vi "RT_Main.vi"() -> ()   [LabVIEW 2019]
uses:
  <vilib>/myRIO/Instrument Drivers/Onboard IO/DIO/typedefs/DIO Reference.ctl
  <vilib>/myRIO/Common/Instrument Driver Framework/Utilities/typedefs/myRIO Generic Hardware Reference.ctl
  <vilib>/myRIO/Common/Instrument Driver Framework/Utilities/typedefs/Hardware Version Enum.ctl
  <vilib>/myRIO/Common/Instrument Driver Framework/Utilities/typedefs/myRIO v1.0 Reference.ctl
  <vilib>/myRIO/Common/Instrument Driver Framework/Utilities/typedefs/Generic FPGA Reference.ctl
  <vilib>/myRIO/Common/Instrument Driver Framework/myRIO v1.0/DIO/typedefs/DIO Channels List.ctl
  <vilib>/myRIO/Common/Instrument Driver Framework/myRIO v1.0/DIO/typedefs/DIO Channels Enum.ctl
  <vilib>/userdefined/High Color/nirio_resource_hc.ctl
  <vilib>/myRIO/Instrument Drivers/Onboard IO/I2C/typedefs/I2C User Configuration.ctl
  <vilib>/myRIO/Instrument Drivers/Onboard IO/I2C/typedefs/I2C Transfer Rate.ctl
  <vilib>/myRIO/Instrument Drivers/Onboard Devices/Accelerometer/typedefs/Accelerometer Reference.ctl
  <vilib>/myRIO/Common/Instrument Driver Framework/myRIO v1.0/Accelerometer/typedefs/Accelerometer Channels List.ctl
  <vilib>/myRIO/Common/Instrument Driver Framework/myRIO v1.0/Accelerometer/typedefs/Accelerometer Channels Enum.ctl
  <vilib>/myRIO/Common/Instrument Driver Framework/Utilities/vis/Is FPGA Ref Available.vi
  <vilib>/myRIO/Common/Instrument Driver Framework/myRIO v1.0/DIO/vis/myRIO v1.1 Open DIO.vi
  <vilib>/myRIO/Common/Instrument Driver Framework/myRIO v1.0/Accelerometer/vis/myRIO v1.1 Open Accelerometer.vi
  <vilib>/myRIO/Common/Instrument Driver Framework/Utilities/vis/Validate Channels.vi
  <vilib>/myRIO/Common/Instrument Driver Framework/myRIO v1.0/DIO/vis/myRIO v1.0 Reserve DIO.vi
  <vilib>/myRIO/Common/Instrument Driver Framework/myRIO v1.0/I2C/vis/myRIO v1.0 Close I2C.vi
  <vilib>/myRIO/Common/Instrument Driver Framework/myRIO v1.0/Accelerometer/vis/myRIO v1.0 Reserve Accelerometer.vi
  <vilib>/myRIO/Common/Instrument Driver Framework/myRIO v1.0/UART/vis/myRIO v1.0 Close UART.vi
  <vilib>/myRIO/Common/Instrument Driver Framework/myRIO v1.0/Resource Manager/vis/myRIO v1.0 Reserve Channel List.vi
  <vilib>/myRIO/Common/Instrument Driver Framework/myRIO v1.0/DIO/vis/myRIO v1.0 Build MUX Configuration DIO.vi
  <vilib>/myRIO/Common/Instrument Driver Framework/myRIO v1.0/I2C/vis/myRIO v1.0 Unreserve I2C.vi
  <vilib>/myRIO/Common/Instrument Driver Framework/myRIO v1.0/Accelerometer/vis/myRIO v1.0 Build MUX Configuration Accelerometer.vi
  <vilib>/myRIO/Common/Instrument Driver Framework/myRIO v1.0/Resource Manager/vis/myRIO v1.0 Reserve Channel.vi
  <vilib>/myRIO/Common/Instrument Driver Framework/myRIO v1.0/Resource Manager/vis/myRIO v1.0 Unreserve Channel.vi
  <vilib>/myRIO/Common/Instrument Driver Framework/myRIO v1.0/Resource Manager/vis/myRIO v1.0 Create Configuration List.vi
  <vilib>/myRIO/Common/Instrument Driver Framework/myRIO v1.0/I2C/vis/myRIO v1.0 Build MUX Configuration I2C.vi
  <vilib>/myRIO/Common/Instrument Driver Framework/myRIO v1.0/Resource Manager/vis/myRIO v1.0 Unreserve Channel List.vi
  <vilib>/myRIO/Common/Instrument Driver Framework/myRIO v1.0/Resource Manager/vis/myRIO v1.0 Build Mutex Name.vi
  <vilib>/functionblocks/Counter/Elapsed Timer/Elapsed Timer.vi
  <vilib>/Utility/VariantDataType/GetNumericInfo.vi
  <vilib>/Utility/error.llb/Error Cluster From Error Code.vi
  <vilib>/myRIO/Common/Instrument Driver Framework/myRIO v1.0/myRIO v1.1 Open.vi
  <vilib>/myRIO/Common/Instrument Driver Framework/Utilities/vis/IO Manager.vi
  <vilib>/myRIO/Common/Instrument Driver Framework/Utilities/vis/Configuration Manager.vi
  <vilib>/myRIO/Common/Instrument Driver Framework/myRIO v1.0/Resource Manager/vis/myRIO v1.0 Configure IO.vi
  <vilib>/myRIO/Common/Instrument Driver Framework/myRIO v1.0/myRIO v1.0 Close.vi
  <vilib>/myRIO/Common/Instrument Driver Framework/myRIO v1.0/DIO/vis/myRIO v1.0 Read DIO.vi
  <vilib>/myRIO/Common/Instrument Driver Framework/myRIO v1.0/PWM/vis/myRIO v1.0 Write PWM.vi
  <vilib>/myRIO/Common/Instrument Driver Framework/myRIO v1.0/DIO/vis/myRIO v1.0 Write DIO.vi
  <vilib>/myRIO/Common/Instrument Driver Framework/myRIO v1.0/Accelerometer/vis/myRIO v1.0 Get Scaling Constant Accelerometer.vi
  <vilib>/myRIO/Common/Instrument Driver Framework/myRIO v1.0/Accelerometer/vis/myRIO v1.0 Read Accelerometer.vi
  <vilib>/myRIO/Common/Instrument Driver Framework/myRIO v1.0/I2C/vis/myRIO v1.0 Configure I2C.vi
  <vilib>/myRIO/Common/Instrument Driver Framework/myRIO v1.0/I2C/vis/myRIO v1.0 Shutdown I2C.vi
  <vilib>/myRIO/Common/Instrument Driver Framework/myRIO v1.0/AI/vis/myRIO v1.0 Read AI.vi
  <vilib>/myRIO/Common/Instrument Driver Framework/Utilities/vis/FPGA Ref Manager.vi
  <vilib>/myRIO/Common/Instrument Driver Framework/myRIO v1.0/myRIO v1.0 Reset FPGA.vi
  <vilib>/myRIO/Common/Instrument Driver Framework/myRIO v1.0/IRQ/vis/myRIO v1.0 IRQ Info FGV.vi
  <vilib>/myRIO/Common/Instrument Driver Framework/myRIO v1.0/IRQ/vis/myRIO v1.0 Timer IRQ Info FGV.vi
  <vilib>/myRIO/Common/Instrument Driver Framework/myRIO v1.0/IRQ/vis/myRIO v1.0 ISR Agent.vi
  <vilib>/myRIO/Instrument Drivers/Utilities/vis/Reset Index.vi
  <vilib>/myRIO/Common/Instrument Driver Framework/myRIO v1.0/Resource Manager/vis/myRIO v1.0 Block Write Resource Manager.vi
  <vilib>/functionblocks/FB Core/FB Core.xnode
  <vilib>/myRIO/Express VI/Onboard IO/DI/DI Express VI.xnode
  <vilib>/myRIO/Instrument Drivers/Onboard IO/DIO/vis/myRIO DIO Open.xnode
  <vilib>/myRIO/Express VI/Onboard Devices/Accelerometer/Accelerometer Express VI.xnode
  <vilib>/myRIO/Instrument Drivers/Onboard Devices/Accelerometer/vis/myRIO Accelerometer Open.xnode
  <vilib>/myRIO/Express VI/Onboard IO/DO/DO Express VI.xnode
  <vilib>/myRIO/Instrument Drivers/Onboard IO/I2C/I2C.lvlib
  <vilib>/myRIO/Instrument Drivers/Onboard IO/AI/AI.lvlib
  <vilib>/myRIO/Instrument Drivers/Utilities/Utilities.lvlib
  <vilib>/functionblocks/NI_FunctionBlock Libraries.lvlib
  <vilib>/myRIO/Instrument Drivers/Onboard IO/DIO/DIO.lvlib
  <vilib>/myRIO/Instrument Drivers/Onboard IO/PWM/PWM.lvlib
  <vilib>/myRIO/Instrument Drivers/Onboard Devices/Accelerometer/Accelerometer.lvlib
panel:
  out "Time":dbl
  out "X-Axis":dbl=-0.00390625
  out "Y-Axis":dbl=-0.1171875
  out "Z-Axis":dbl=0.98046875
  in  "Tab Control":T1(tab)
  out "Cluster":T2
  in  "Tab Control 3":enum32{"Simple", "Advanced"}(tab)
  in  "Up Button":bool
  in  "Down Button":bool
  in  "Enable":bool
  in  "Direction":bool
  out "Accelerometer Readings":T2(graph)={"X-Axis"=-0.00390625, "Y-Axis"=-0.1171875, "Z-Axis"=0.98046875}
  out "GPS Time":string
  in  "Air Sample":bool
  in  "Log File Name":string="LocationLog"
  in  "Sampler Step Freq":dbl(slide)=253.06122448979593 scale=100.0..300.0
  out "Storage Status":string=" 34.4 GB capacity with 25.7 GB free (74.8%)"
  in  "Plot Reset":bool
  out "Latitude":dbl=0.03333333333333333
  out "Longitude":dbl=0.050000555555555555
  out "Speed":dbl
  out "GPS Location":cluster{dbl[], dbl[]}(graph)
  out "IR Distance Left":dbl=740.0516187067414 format="%#3_4g"
  out "IR Distance Right":dbl=1850.783507510213 format="%#_4g"
  out "Sonar Distance":dbl=80.530998125 format="%#_4g"
  in  "Stop button":bool
  in  "Log Data?":bool=TRUE
  out "Logging Error Out":errorcluster
  out "File storage error out":errorcluster
  out "error IO":errorcluster
  out "Accelerometer Error Out":errorcluster
  out "Initialize Error Out":errorcluster={"status"=FALSE, "code"=-1950679034, "source"="Shared Variable in RT_Main.vi<APPEND>\nThis error or warning occurred while reading the following Shared Variable:\n\\\\OSoleRIO\\Target Library\\SonarDistance\n\\\\172.16.0.1\\Target Library\\SonarDistance"}
  out "Initialization Timed Out?":bool
  out "Main":i32=272259
  out "GPS":i32=1046
  out "IR":i32=5434
  out "Sonar":i32=2765
  out "UI":i32=25031
  out "Motor":i32=299489
  out "Logging":i32=126701
  out "Storage Status 2":i32=558
  out "Accelerometer":i32
  in  "Time zone":i32=1
  # "Soil Sample"
  # "True=Up False=Down"
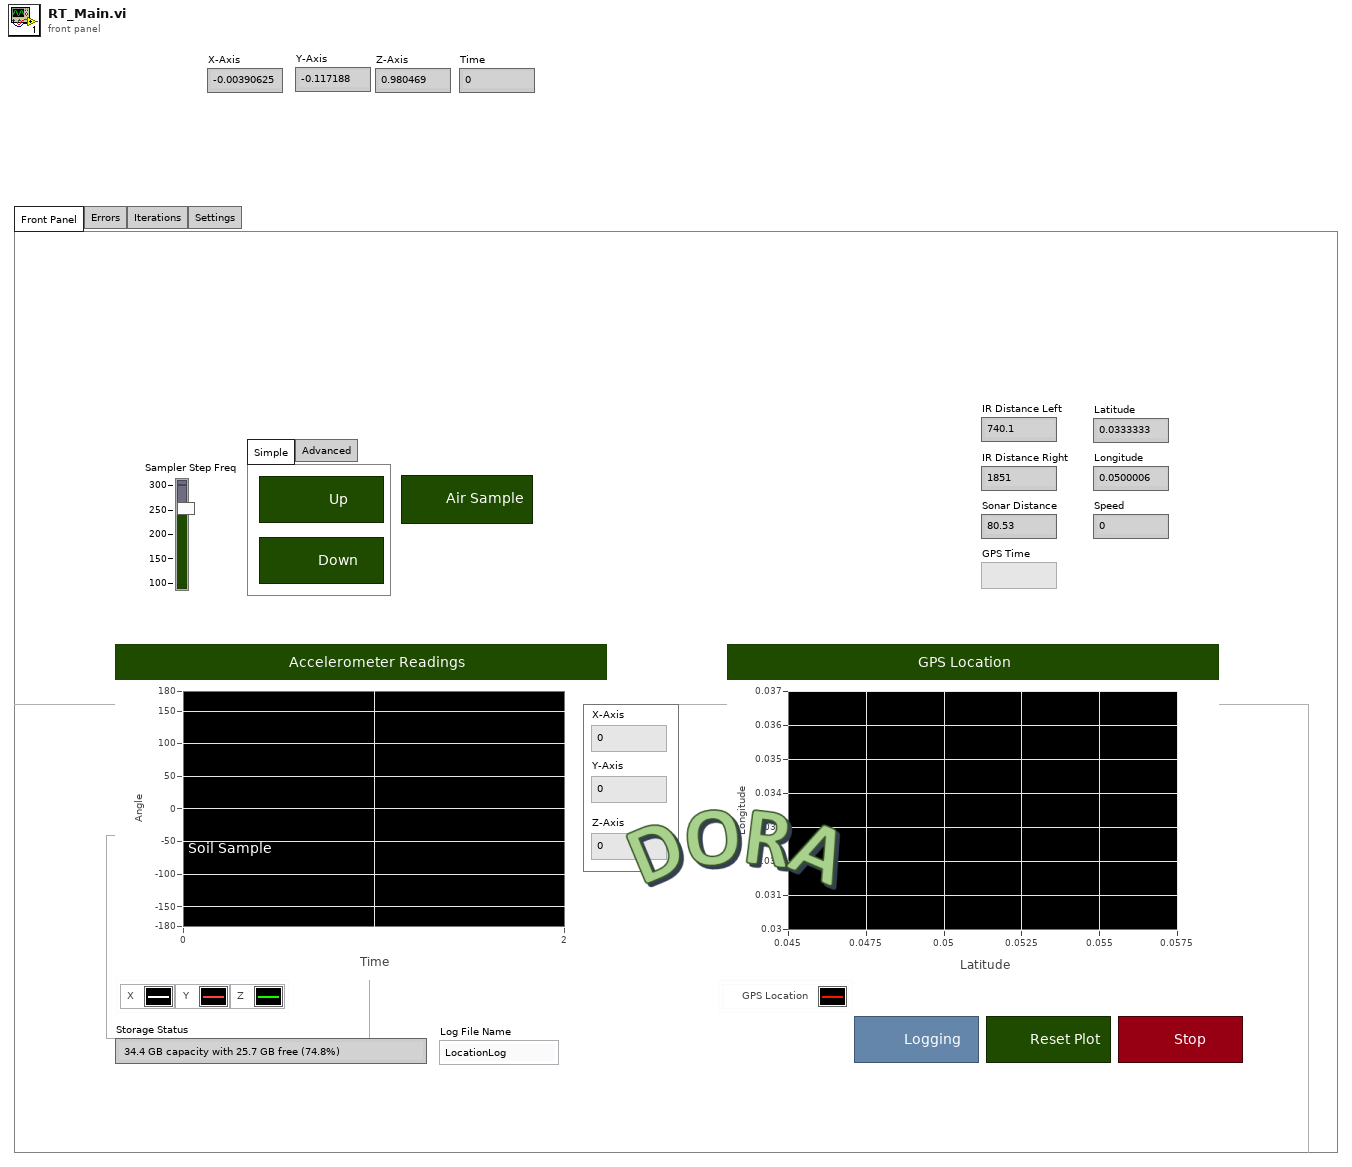
[diagram p1: front panel]
types:
  T1 = enum32{"Front Panel", "Errors", "Iterations", "Settings"}
  T2 = cluster{"X-Axis":dbl, "Y-Axis":dbl, "Z-Axis":dbl}
  T3 = enum16{"open", "replace", "create", "open or create", "replace or create", "replace or create with confirmation"}
  T4 = typedef "DIO.lvlib/DIO Reference.ctl" = cluster{"myRIO Reference":T5, "DIO Channels List":T9}
  T5 = typedef "myRIO Generic Hardware Reference.ctl" = cluster{"myRIO Model":T6, "myRIO Hardware Reference":T7}
  T6 = typedef "Hardware Version Enum.ctl" = enum16{"Unknown", "myRIO-1900", "myRIO-1950", "roboRIO", "NI ELVIS RIO CM", "ELVIS III"}
  T7 = typedef "myRIO v1.0 Reference.ctl" = cluster{"Generic FPGA Reference":T8, "Allow multiple opens":bool}
  T8 = typedef "Generic FPGA Reference.ctl" = refnum<k20>
  T9 = typedef "DIO Channels List.ctl" = T10[]
  T10 = typedef "DIO Channels Enum.ctl" = enum16{"Not Connected", "C/DIO0", "C/DIO1", "C/DIO2", "C/DIO3", "C/DIO4", "C/DIO5", "C/DIO6", "C/DIO7", "A/DIO0", "A/DIO1", "A/DIO2", "A/DIO3", "A/DIO4", "A/DIO5", "A/DIO6", "A/DIO7", "A/DIO8", "A/DIO9", "A/DIO10", "A/DIO11", "A/DIO12", "A/DIO13", "A/DIO14", "A/DIO15", "A/DIO16", "A/DIO17", "A/DIO18", "A/DIO19", "B/DIO0", "B/DIO1", "B/DIO2", "B/DIO3", "B/DIO4", "B/DIO5", "B/DIO6", "B/DIO7", "B/DIO8", "B/DIO9", "B/DIO10", "B/DIO11", "B/DIO12", "B/DIO13", "B/DIO14", "B/DIO15", "B/DIO16", "B/DIO17", "B/DIO18", "B/DIO19", "LED0", "LED1", "LED2", "LED3", "Button0", "DIO/DIO0", "DIO/DIO1", "DIO/DIO2", "DIO/DIO3", "DIO/DIO4", "DIO/DIO5", "DIO/DIO6", "DIO/DIO7", "DIO/DIO8", "DIO/DIO9", "SPI/CS0", "SPI/CS1", "SPI/CS2", "SPI/CS3", "LED RADIO (Green)", "LED RADIO (Red)", "LED COMM (Green)", "LED COMM (Red)", "LED MODE (Green)", "LED MODE (Red)"}
  T11 = typedef "nirio_resource_hc.ctl" = tag
  T12 = typedef "I2C.lvlib/I2C User Configuration.ctl" = cluster{"I2C Transfer Rate":T13}
  T13 = typedef "I2C.lvlib/I2C Transfer Rate.ctl" = enum16{"Standard mode (100 kbps)", "Fast mode (400 kbps)"}
  T14 = typedef "Accelerometer.lvlib/Accelerometer Reference.ctl" = cluster{"myRIO Reference":T5, "Accelerometer Channels List":T15, "LSB Weight":dbl}
  T15 = typedef "Accelerometer Channels List.ctl" = T16[]
  T16 = typedef "Accelerometer Channels Enum.ctl" = enum16{"Not Connected", "X-Axis", "Y-Axis", "Z-Axis"}
  T17 = typedef "AI.lvlib/AI Reference.ctl" = cluster{"myRIO Reference":T5, "AI Channels List":T18, "AI Scaling Constants List":T20}
  T18 = typedef "AI Channels List.ctl" = T19[]
  T19 = typedef "AI Channels Enum.ctl" = enum16{"Not Connected", "AudioIn/Left", "AudioIn/Right", "C/AI0", "C/AI1", "A/AI0", "A/AI1", "A/AI2", "A/AI3", "A/AI4", "A/AI5", "A/AI6", "A/AI7", "B/AI0", "B/AI1", "B/AI2", "B/AI3", "B/AI4", "B/AI5", "B/AI6", "B/AI7", "AI/AI0", "AI/AI1", "AI/AI2", "AI/AI3", "A/AI0 (DIFF)", "A/AI1 (DIFF)", "A/AI2 (DIFF)", "A/AI3 (DIFF)", "B/AI0 (DIFF)", "B/AI1 (DIFF)", "B/AI2 (DIFF)", "B/AI3 (DIFF)"}
  T20 = typedef "Analog Scaling Constants List.ctl" = T21[]
  T21 = typedef "Analog Scaling Constants.ctl" = cluster{"LSB Weight (Volts)":dbl, "Offset (Volts)":dbl, "Signed?":bool}
  T22 = typedef "PWM.lvlib/PWM Reference.ctl" = cluster{"myRIO Reference":T5, "PWM Channels Enum":T23, "PWM Configuration":T24}
  T23 = typedef "PWM Channels Enum.ctl" = enum16{"Not Connected", "C/PWM0", "C/PWM1", "A/PWM0", "A/PWM1", "A/PWM2", "A/PWM3", "A/PWM4", "A/PWM5", "A/PWM6", "A/PWM7", "A/PWM8", "A/PWM9", "A/PWM10", "A/PWM11", "A/PWM12", "A/PWM13", "A/PWM14", "A/PWM15", "A/PWM16", "A/PWM17", "A/PWM18", "A/PWM19", "B/PWM0", "B/PWM1", "B/PWM2", "B/PWM3", "B/PWM4", "B/PWM5", "B/PWM6", "B/PWM7", "B/PWM8", "B/PWM9", "B/PWM10", "B/PWM11", "B/PWM12", "B/PWM13", "B/PWM14", "B/PWM15", "B/PWM16", "B/PWM17", "B/PWM18", "B/PWM19", "PWM/PWM0", "PWM/PWM1", "PWM/PWM2", "PWM/PWM3", "PWM/PWM4", "PWM/PWM5", "PWM/PWM6", "PWM/PWM7", "PWM/PWM8", "PWM/PWM9"}
  T24 = typedef "PWM.lvlib/PWM Configuration.ctl" = cluster{"Frequency":dbl, "Duty Cycle":dbl}
  T25 = typedef "I2C.lvlib/I2C Reference.ctl" = cluster{"myRIO Reference":T5, "I2C Channels Enum":T26, "I2C Configuration":T27}
  T26 = typedef "I2C Channels Enum.ctl" = enum16{"Not Connected", "A/I2C", "B/I2C", "I2C/I2C"}
  T27 = typedef "I2C.lvlib/I2C Configuration.ctl" = cluster{"I2C Transfer Rate":T13}
  T28 = cluster{"Time String":string, "Time Value":dbl, "Latitude":dbl, "Longitude":dbl, "Speed [m/s]":dbl}
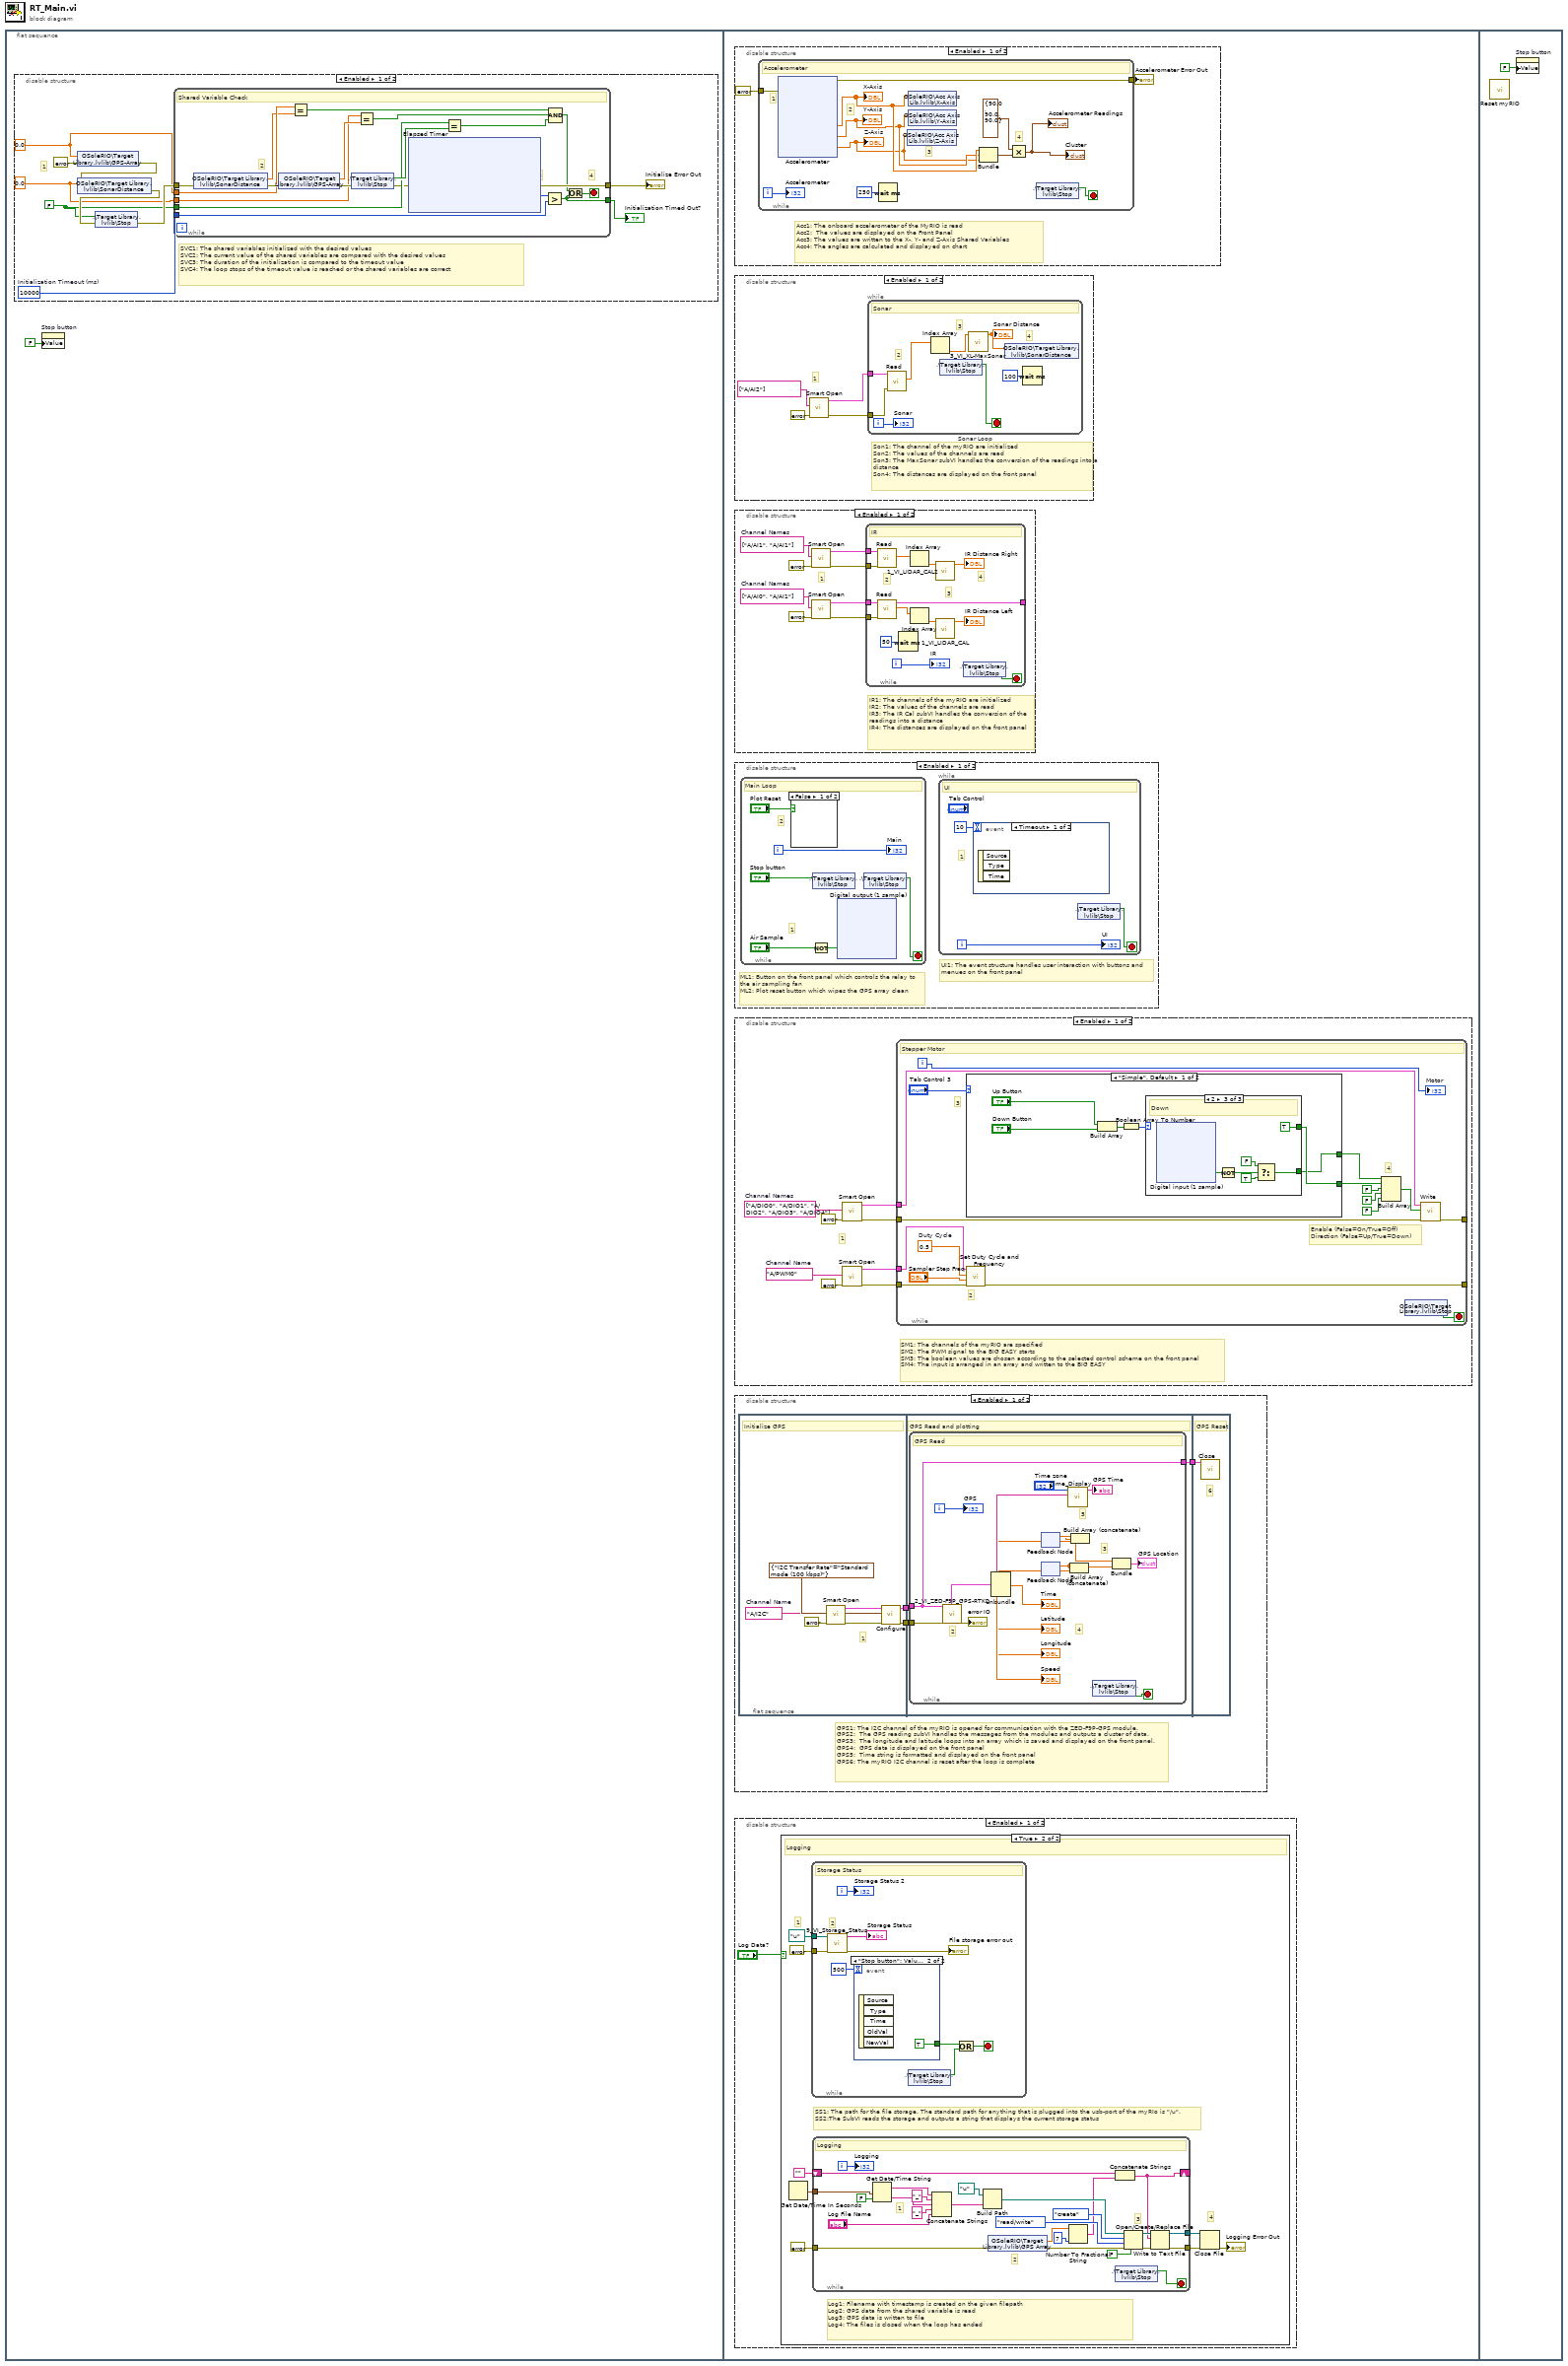
[diagram p0: block diagram]
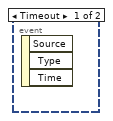
[diagram p5: hidden frame]
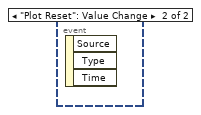
[diagram p7: hidden frame]
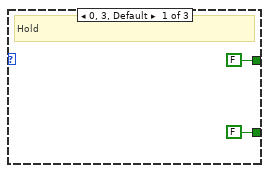
[diagram p13: hidden frame]
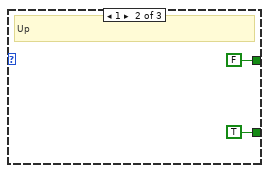
[diagram p14: hidden frame]
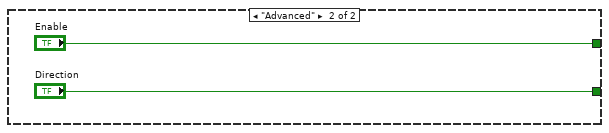
[diagram p15: hidden frame]
diagram:
  n1 = flat-sequence {
    frame #0 {
      n2 = disable-structure shown="Enabled" {
        frame Enabled {
          w3 = 10000  # Initialization Timeout (ms)
          w5 = 0.0 ("SonarDistance")
          w6 = 0.0 ("GPS-Array")
          w7 = FALSE ("Stop")
          # "1"
          # "SVC1: The shared variables initialized with the desired values \nSVC2: The current value of the shared variables are compared with the desired values\nSVC3: The duration of the initialization is compared to the timeout value\nSVC4: The loop stops of the timeout value is reached or the shared variables are correct"
          n3 = shared-variable "OSoleRIO\\Target Library.lvlib\\GPS-Array"(w6, error in=errorcluster {"status"=FALSE, "code"=0, "source"=""} ("error in (no error)")) -> (error out=w10:errorcluster)
          n4 = shared-variable "OSoleRIO\\Target Library.lvlib\\SonarDistance"(w5, error in=w10) -> (error out=w9:errorcluster)
          n5 = shared-variable ".\\Target Library.lvlib\\Stop"(w7, error in=w9) -> (error out=w8:errorcluster)
          n6 = while {
            tunnel: w8 -> [w30]
            tunnel: w7 -> [w26]
            tunnel: w6 -> [w22]
            tunnel: w5 -> [w20]
            tunnel: [w17] -> w4
            tunnel: w3 -> [w14]
            tunnel: [w12] -> w2
            stop <- w13 stop-if-true
            # "4"
            # "3"
            # "2"
            # "Shared Variable Check"
            n7 = shared-variable "OSoleRIO\\Target Library.lvlib\\SonarDistance"(error in=w30) -> (w19:dbl, error out=w29:errorcluster)
            n8 = shared-variable "OSoleRIO\\Target Library.lvlib\\GPS-Array"(error in=w29) -> (w21:dbl, error out=w28:errorcluster)
            n9 = Equal?(x=w22, y=w19) -> (x = y?=w23:bool)
            n10 = shared-variable ".\\Target Library.lvlib\\Stop"(error in=w28) -> (w27:bool, error out=w18:errorcluster)
            n11 = Equal?(x=w20, y=w21) -> (x = y?=w24:bool)
            n12 = xnode "Elapsed Timer"("error in"=w18) -> ("error out"=w17:errorcluster, "elapsed time (ms)"=w15:i32)  [unwired: 2 in]
            n13 = Equal?(x=w26, y=w27) -> (x = y?=w25:bool)
            n14 = Greater?(x=w15, y=w14) -> (0:w12:bool)
            n15 = Compound Arithmetic op=AND(w23, w24, w25) -> (w16:bool)
            n16 = Or(x=w16, y=w12) -> (x .or. y?=w13:bool)
          }
          "Initialize Error Out" <- w4
          "Initialization Timed Out?" <- w2
        }
        frame Disabled {
        }
      }
      n17 = property on="Stop button" class="Bool (strict)"("Value"=FALSE ("Stop")) -> ()  [unwired: 2 in, 2 out]
    }
    frame #1 {
      n18 = disable-structure shown="Enabled" {
        frame Enabled {
          # "Acc1: The onboard accelerometer of the MyRIO is read\nAcc2:  The values are displayed on the Front Panel\nAcc3: The values are written to the X-, Y- and Z-Axis Shared Variables\nAcc4: The angles are calculated and displayed on chart"
          n19 = while {
            tunnel: [w232] -> w222
            tunnel: errorcluster {"status"=FALSE, "code"=0, "source"=""} ("error in (no error)") -> [w231]
            i -> [w225]
            stop <- w230 stop-if-true
            # "4"
            # "3"
            # "2"
            # "1"
            # "Accelerometer"
            n20 = xnode "Accelerometer"("error in (no error)"=w231) -> ("X-Axis"=w229:dbl, "Y-Axis"=w228:dbl, "Z-Axis"=w227:dbl, "error out"=w232:errorcluster)
            "X-Axis" <- w229
            "Y-Axis" <- w228
            "Z-Axis" <- w227
            n21 = Wait (ms)(milliseconds to wait=u32 250) -> ()  [unwired: 1 out]
            n22 = shared-variable "OSoleRIO\\Acc Axis Lib.lvlib\\Z-Axis"(w227) -> ()  [unwired: 1 in, 1 out]
            n23 = shared-variable "OSoleRIO\\Acc Axis Lib.lvlib\\X-Axis"(w229) -> ()  [unwired: 1 in, 1 out]
            n24 = shared-variable "OSoleRIO\\Acc Axis Lib.lvlib\\Y-Axis"(w228) -> ()  [unwired: 1 in, 1 out]
            n25 = Bundle("X-Axis"=w229, "Y-Axis"=w228, "Z-Axis"=w227) -> (w226:T2)  [unwired: 1 in]
            n26 = Multiply(x=T2 {"X-Axis"=90.0, "Y-Axis"=90.0, "Z-Axis"=90.0}, y=w226) -> (x*y=→"Accelerometer Readings" →"Cluster":T2)
            n27 = shared-variable ".\\Target Library.lvlib\\Stop"() -> (w230:bool)  [unwired: 1 in, 1 out]
            "Accelerometer" <- w225
          }
          "Accelerometer Error Out" <- w222
        }
        frame Disabled {
        }
      }
      n28 = disable-structure shown="Enabled" {
        frame Enabled {
          # "Son1: The channel of the myRIO are initialized \nSon2: The values of the channels are read \nSon3: The MaxSonar subVI handles the conversion of the readings into a distance\nSon4: The distances are displayed on the front panel"
          # "1"
          n29 = call <vilib>:"Smart Open.vi"("error in (no error)"=errorcluster {"status"=FALSE, "code"=0, "source"=""}, "Channel Names"=tag[] ["A/AI2"]) -> ("error out"=w67:errorcluster, "AI Ref Out"=w68:T17)  [unwired: 8 in]
          n30 = while "Sonar Loop" {
            tunnel: w68 -> [w76]
            tunnel: w67 -> [w75]
            i -> [w78]
            stop <- w77 stop-if-true
            # "4"
            # "3"
            # "2"
            # "Sonar"
            n31 = call <vilib>:"Read.vi"("error in (no error)"=w75, "AI Ref In"=w76) -> ("Values"=w74:dbl[])  [unwired: 7 in, 2 out]
            n32 = Index Array(array=w74) -> (element=w73:dbl)  [unwired: 1 in]
            n33 = shared-variable ".\\Target Library.lvlib\\Stop"() -> (w77:bool)  [unwired: 1 in, 1 out]
            n34 = call "3_VI_XL-MaxSonar.vi"("Analog IN [V]"=w73) -> ("Sonar Distance"=w71:dbl)  [unwired: 9 in]
            "Sonar Distance" <- w71
            n35 = shared-variable "OSoleRIO\\Target Library.lvlib\\SonarDistance"(w71) -> ()  [unwired: 1 in, 1 out]
            n36 = Wait (ms)(milliseconds to wait=u32 100) -> ()  [unwired: 1 out]
            "Sonar" <- w78
          }
        }
        frame Disabled {
        }
      }
      n37 = disable-structure shown="Enabled" {
        frame Enabled {
          w170 = tag[] ["A/AI1", "A/AI1"]  # Channel Names
          w175 = tag[] ["A/AI0", "A/AI1"]  # Channel Names
          # "1"
          # "IR1: The channels of the myRIO are initialized\nIR2: The values of the channels are read\nIR3: The IR Cal subVI handles the conversion of the readings into a distance\nIR4: The distances are displayed on the front panel"
          n38 = call <vilib>:"Smart Open.vi"("error in (no error)"=errorcluster {"status"=FALSE, "code"=0, "source"=""}, "Channel Names"=w170) -> ("error out"=w168:errorcluster, "AI Ref Out"=w169:T17)  [unwired: 8 in]
          n39 = call <vilib>:"Smart Open.vi"("error in (no error)"=errorcluster {"status"=FALSE, "code"=0, "source"=""}, "Channel Names"=w175) -> ("error out"=w174:errorcluster, "AI Ref Out"=w173:T17)  [unwired: 8 in]
          n40 = while "Sensor Loop" {
            tunnel: w174 -> [w186]
            tunnel: w173 -> [w185]
            tunnel: [w180] -> _
            tunnel: w169 -> [w179]
            tunnel: w168 -> [w178]
            i -> [w188]
            stop <- w189 stop-if-true
            # "4"
            # "3"
            # "2"
            # "IR"
            n41 = call <vilib>:"Read.vi"("error in (no error)"=w178, "AI Ref In"=w179) -> ("Values"=w177:dbl[])  [unwired: 7 in, 2 out]
            n42 = call <vilib>:"Read.vi"("error in (no error)"=w186, "AI Ref In"=w185) -> ("Values"=w184:dbl[], "AI Ref Out"=w180:T17)  [unwired: 7 in, 1 out]
            n43 = Wait (ms)(milliseconds to wait=u32 50) -> ()  [unwired: 1 out]
            n44 = Index Array(array=w177) -> (element=w176:dbl)  [unwired: 1 in]
            n45 = Index Array(array=w184) -> (element=w183:dbl)  [unwired: 1 in]
            n46 = call "1_VI_LIDAR_CAL2.vi"("Analog input"=w176) -> ("LidarDistance"=→"IR Distance Right":dbl)  [unwired: 10 in]
            n47 = call "1_VI_LIDAR_CAL.vi"("Analog input"=w183) -> ("IRDistance"=→"IR Distance Left":dbl)  [unwired: 10 in]
            n48 = shared-variable ".\\Target Library.lvlib\\Stop"() -> (w189:bool)  [unwired: 1 in, 1 out]
            "IR" <- w188
          }
        }
        frame Disabled {
        }
      }
      n49 = disable-structure shown="Enabled" {
        frame Enabled {
          # "UI1: The event structure handles user interaction with buttons and menues on the front panel"
          # "ML1: Button on the front panel which controls the relay to the air sampling fan\nML2: Plot reset button which wipes the GPS array clean"
          n50 = while "Main Loop" {
            i -> [w131]
            stop <- w132 stop-if-true
            # "1"
            # "2"
            # "Main Loop"
            n51 = case shown="False" "Plot Reset" {
              frame False {
              }
              frame True {
              }
            }
            n52 = Not(x="Air Sample") -> (.not. x?=w127:bool)
            n53 = shared-variable ".\\Target Library.lvlib\\Stop"("Stop button") -> ()  [unwired: 1 in, 1 out]
            n54 = xnode "Digital output (1 sample)"("B/DIO13 (Pin 26)"=w127) -> ()  [unwired: 1 in, 1 out]
            n55 = shared-variable ".\\Target Library.lvlib\\Stop"() -> (w132:bool)  [unwired: 1 in, 1 out]
            "Main" <- w131
          }
          n56 = while "UI Loop" {
            i -> [w126]
            stop <- w125 stop-if-true
            # "1"
            # "UI"
            n57 = event shown="[0] Timeout" {
              selector: _ -> [_ _]
              dyn-events: _ -> [_ _]
              timeout: 10 -> [_ _]
              event Timeout {
                n58 = event-data() -> ()  [unwired: 1 in, 3 out]
              }
              event "Plot Reset": Value Change {
                n59 = event-data() -> ()  [unwired: 1 in, 3 out]
              }
            }
            n60 = shared-variable ".\\Target Library.lvlib\\Stop"() -> (w125:bool)  [unwired: 1 in, 1 out]
            "UI" <- w126
          }
        }
        frame Disabled {
        }
      }
      n61 = disable-structure shown="Enabled" {
        frame Enabled {
          w275 = tag[] ["A/DIO0", "A/DIO1", "A/DIO2", "A/DIO3", "A/DIO4"]  # Channel Names
          w279 = tag "A/PWM0"  # Channel Name
          # "1"
          # "SM1: The channels of the myRIO are specified \nSM2: The PWM signal to the BIG EASY starts\nSM3: The boolean values are chosen according to the selected control scheme on the front panel \nSM4: The input is arranged in an array and written to the BIG EASY"
          n62 = call <vilib>:"Smart Open.vi"("error in (no error)"=errorcluster {"status"=FALSE, "code"=0, "source"=""}, "Channel Names"=w275) -> ("error out"=w276:errorcluster, "DIO Ref Out"=w277:T4)  [unwired: 8 in]
          n63 = call <vilib>:"Smart Open.vi"("error in (no error)"=errorcluster {"status"=FALSE, "code"=0, "source"=""} ("error in (no error) 2"), "Channel Name"=w279) -> ("error out"=w280:errorcluster, "PWM Ref Out"=w281:T22)  [unwired: 8 in]
          n64 = while {
            tunnel: w276 -> [w293]
            tunnel: w277 -> [w292]
            tunnel: w280 -> [w291]
            tunnel: w281 -> [w290]
            tunnel: [w289] -> _
            tunnel: [w288] -> _
            i -> [w286]
            stop <- w287 stop-if-true
            w294 = 0.5  # Duty Cycle
            # "4"
            # "3"
            # "2"
            # "Enable (False=On/True=Off)\nDirection (False=Up/True=Down)"
            # "Stepper Motor"
            n65 = case shown="\"Simple\", Default" "Tab Control 3" {
              tunnel: [w300 "Direction"] -> w284
              tunnel: [w299 "Enable"] -> w283
              frame "Simple", Default {
                n66 = Build Array("Up Button", "Down Button") -> (w304:bool[])
                n67 = Boolean Array To Number(Boolean array=w304) -> (number=w303:u32)
                n68 = case shown="2" w303 {
                  tunnel: [FALSE ("element") FALSE ("element") TRUE ("element")] -> w300
                  tunnel: [FALSE ("element") TRUE ("element") w309] -> w299
                  frame 0, 3, Default {
                    # "Hold"
                  }
                  frame 1 {
                    # "Up"
                  }
                  frame 2 {
                    # "Down"
                    n69 = xnode "Digital input (1 sample)"() -> ("B/DIO7 (Pin 25)"=w311:bool)  [unwired: 1 in, 1 out]
                    n70 = Not(x=w311) -> (.not. x?=w310:bool)
                    n71 = Select(t=FALSE, s=w310, f=TRUE ("element")) -> (s? t:f=w309:bool)
                  }
                }
              }
              frame "Advanced" {
              }
            }
            n72 = call <vilib>:"Set Duty Cycle and Frequency.vi"("error in (no error)"=w291, "Frequency [Hz]"="Sampler Step Freq", "Duty Cycle"=w294, "PWM Ref In"=w290) -> ("error out"=w288:errorcluster)  [unwired: 5 in, 1 out]
            n73 = Build Array(w283, w284, FALSE ("MS1 (A/DIO2 (Pin 15))"), FALSE ("MS2 (A/DIO3 (Pin 17))"), FALSE ("MS3 (A/DIO4 (Pin 19))")) -> (w298:bool[])
            n74 = shared-variable "OSoleRIO\\Target Library.lvlib\\Stop"() -> (w287:bool)  [unwired: 1 in, 1 out]
            n75 = call <vilib>:"Write.vi"("error in (no error)"=w293, "Values"=w298, "DIO Ref In"=w292) -> ("error out"=w289:errorcluster)  [unwired: 6 in, 1 out]
            "Motor" <- w286
          }
        }
        frame Disabled {
        }
      }
      n76 = disable-structure shown="Enabled" {
        frame Enabled {
          # "GPS1: The I2C channel of the myRIO is opened for communication with the ZED-F9P-GPS module. \nGPS2:  The GPS reading subVI handles the messages from the modules and outputs a cluster of data.\nGPS3:  The longitude and latitude loops into an array which is saved and displayed on the front panel.\nGPS4:  GPS data is displayed on the front panel \nGPS5:  Time string is formatted and displayed on the front panel\nGPS6: The myRIO I2C channel is reset after the loop is complete"
          n77 = flat-sequence {
            tunnel: [w195] -> w192
            tunnel: [w194] -> w191
            tunnel: w192 -> [w202]
            tunnel: w191 -> [w201]
            tunnel: [w200] -> w190
            tunnel: w190 -> [w221]
            frame #0 {
              w196 = tag "A/I2C"  # Channel Name
              # "1"
              # "Initialize GPS"
              n78 = call <vilib>:"Smart Open.vi"("error in (no error)"=errorcluster {"status"=FALSE, "code"=0, "source"=""}, "Channel Name"=w196) -> ("error out"=w199:errorcluster, "I2C Ref Out"=w198:T25)  [unwired: 8 in]
              n79 = call <vilib>:"Configure.vi"("error in (no error)"=w199, "I2C User Configuration"=T12 {"I2C Transfer Rate"=enum."Standard mode (100 kbps)"}, "I2C Ref In"=w198) -> ("error out"=w194:errorcluster, "I2C Ref Out"=w195:T25)  [unwired: 7 in]
            }
            frame #1 {
              # "GPS Read and plotting"
              n80 = while "GPS Loop" {
                tunnel: w202 -> [w207]
                tunnel: w201 -> [w208]
                tunnel: [w207] -> w200
                i -> [w216]
                stop <- w220 stop-if-true
                # "5"
                # "4"
                # "3"
                # "2"
                # "GPS Read"
                n81 = call "2_VI_ZED-F9P_GPS-RTK2.vi"("I2C Ref In"=w207, "error in (no error)"=w208) -> ("output cluster"=w215:T28, "error IO"=→"error IO":errorcluster)  [unwired: 16 in]
                n82 = Unbundle(w215) -> ("Time String"=w214:string, "Time Value"=→"Time":dbl, "Latitude"=w212:dbl, "Longitude"=w211:dbl, "Speed [m/s]"=→"Speed":dbl)
                "Latitude" <- w212
                "Longitude" <- w211
                n83 = feedback #1() -> (w217:dbl[])  [unwired: 1 in]
                n84 = feedback #2() -> (w218:dbl[])  [unwired: 1 in]
                n85 = call "Time_Display.vi"("Time Value"=w214, "Time zone"="Time zone") -> ("Time"=→"GPS Time":string)  [unwired: 9 in]
                n86 = Build Array (concatenate)(w218, w212) -> (w205:dbl[])
                n87 = feedback-in #2(w205) -> ()
                n88 = Build Array (concatenate)(w217, w211) -> (w206:dbl[])
                n89 = feedback-in #1(w206) -> ()
                n90 = shared-variable ".\\Target Library.lvlib\\Stop"() -> (w220:bool)  [unwired: 1 in, 1 out]
                n91 = Bundle(w206, w205) -> (→"GPS Location":cluster{dbl[], dbl[]})  [unwired: 1 in]
                "GPS" <- w216
              }
            }
            frame #2 {
              # "6"
              # "GPS Reset"
              n92 = call <vilib>:"Close.vi"("I2C Ref In"=w221) -> ()  [unwired: 10 in, 1 out]
            }
          }
        }
        frame Disabled {
        }
      }
      n93 = disable-structure shown="Enabled" {
        frame Enabled {
          n94 = case "Logging Case Structure" shown="True" "Log Data?" {
            frame False {
            }
            frame True {
              # "4"
              # "Log1: Filename with timestamp is created on the given filepath\nLog2: GPS data from the shared variable is read\nLog3: GPS data is written to file\nLog4: The files is closed when the loop has ended"
              # "1"
              # "SS1: The path for the file storage. The standard path for anything that is plugged into the usb-port of the myRIo is \"/u\".\nSS2:The SubVI reads the storage and outputs a string that displays the current storage status"
              # "Logging"
              n95 = Get Date/Time In Seconds() -> (seconds since 1Jan1904=w80:timestamp)
              n96 = while {
                tunnel: errorcluster {"status"=FALSE, "code"=0, "source"=""} ("error in") -> [w94]
                tunnel: path "u:/" -> [w89]
                i -> [w95]
                stop <- w90 stop-if-true
                # "2"
                # "Storage Status"
                n97 = call "9_VI_Storage_Status.vi"("error in"=w94, "File Path Control"=w89) -> ("File storage error out"=→"File storage error out":errorcluster, "Storage Status"=→"Storage Status":string)  [unwired: 8 in]
                n98 = event shown="[1] \"Stop button\": Value Change" {
                  selector: _ -> [_ _]
                  dyn-events: _ -> [_ _]
                  timeout: 500 -> [_ _]
                  tunnel: [_ TRUE] -> w91
                  event Timeout {
                    n99 = event-data() -> ()  [unwired: 1 in, 3 out]
                  }
                  event "Stop button": Value Change {
                    n100 = event-data() -> ()  [unwired: 1 in, 5 out]
                  }
                }
                n101 = shared-variable ".\\Target Library.lvlib\\Stop"() -> (w92:bool)  [unwired: 1 in, 1 out]
                n102 = Or(x=w91, y=w92) -> (x .or. y?=w90:bool)
                "Storage Status 2" <- w95
              }
              n103 = while "Logging Loop" {
                tunnel: errorcluster {"status"=FALSE, "code"=0, "source"=""} ("error in") -> [w101]
                shift-right: [w105] -> _
                shift-left: "" -> [w107]
                tunnel: [w110] -> w84
                tunnel: [w109] -> w83
                tunnel: w80 -> [w98]
                i -> [w113]
                stop <- w123 stop-if-true
                # "3"
                # "2"
                # "1"
                # "Logging"
                n104 = Get Date/Time String(seconds (now)=w98, want seconds? (F)=FALSE) -> (date string=w104:string, time string=w103:string)  [unwired: 1 in]
                n105 = Concatenate Strings(w104, "_" ("string"), w103, "_" ("string"), "Log File Name") -> (w118:string)
                n106 = Build Path(base path=path "u:/", name or relative path=w118) -> (appended path=w119:path)
                n107 = shared-variable "OSoleRIO\\Target Library.lvlib\\GPS Array"(error in=w101) -> (w99:dbl[], error out=w100:errorcluster)
                n108 = Number To Fractional String(number=w99, precision (6)=i16 7) -> (F-format string=w106:string[])  [unwired: 2 in]
                n109 = shared-variable ".\\Target Library.lvlib\\Stop"() -> (w123:bool)  [unwired: 1 in, 1 out]
                n110 = Concatenate Strings(w107, w106) -> (w105:string)
                n111 = Open/Create/Replace File(file path (use dialog)=w119, error in=w100, operation (0:open)=T3."create", access (0:read/write)=enum16{"read/write", "read-only", "write-only"}."read/write", disable buffering (F)=FALSE) -> (refnum out=w112:refnum<file>, error out=w111:errorcluster)  [unwired: 1 in, 1 out]
                n112 = Write to Text File(file (use dialog)=w112, text=w105, error in=w111) -> (refnum out=w109:refnum<file>, error out=w110:errorcluster)  [unwired: 1 in, 1 out]
                "Logging" <- w113
              }
              n113 = Close File(refnum=w83, error in=w84) -> (error out=→"Logging Error Out":errorcluster)  [unwired: 1 out]
            }
          }
        }
        frame Disabled {
        }
      }
    }
    frame #2 {
      n114 = call <vilib>:"Reset myRIO.vi"() -> ()  [unwired: 11 in, 1 out]
      n115 = property on="Stop button" class="Bool (strict)"("Value"=FALSE ("Stop")) -> ()  [unwired: 2 in, 2 out]
    }
  }
